vi "SetupDialog.vi"(8 "error in (no error)":errorcluster, 11 "Cluster in":T1 {"frequency" format="%0.2p"; "amplitude" format="%0.2p"; "phase" format="%.2p"; "sampling info"."Fs" format="%.2p"; "square wave duty cycle (%)" format="%0.2f"; "offset" format="%0.2p"}) -> (0 "error out":errorcluster, 3 "Cluster out":T1 {"frequency" format="%0.2p"; "amplitude" format="%0.2p"; "phase" format="%.2p"; "sampling info"."Fs" format="%.2p"; "square wave duty cycle (%)" format="%0.2f"; "offset" format="%0.2p"})   [LabVIEW 2022 SP3]
uses:
  MainBuf.ctl
panel:
  in  "frequency":dbl=10.0 format="%0.2p"
  in  "amplitude":dbl=1.0 format="%0.2p"
  in  "phase":dbl format="%.2p"
  in  "signal type":T2(ring)
  in  "sampling info":cluster{"Fs":dbl, "#s":dbl}={"Fs"=1024.0, "#s"=1024.0} {"Fs" format="%.2f"}
  in  "square wave duty cycle (%)":dbl=50.0 format="%0.2f"
  in  "offset":dbl format="%0.2p"
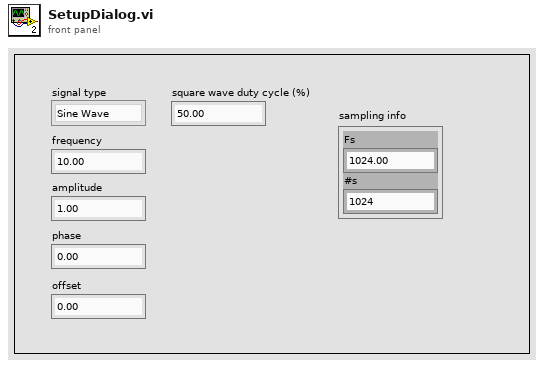
[diagram p1: front panel]
types:
  T1 = typedef "MainBuf.ctl" = cluster{"signal type":enum16{"Sine Wave", "Triangle Wave", "Square Wave", "Sawtooth Wave"}, "frequency":dbl, "amplitude":dbl, "phase":dbl, "offset":dbl, "square wave duty cycle (%)":dbl, "sampling info":cluster{"Fs":dbl, "#s":dbl}, "Reset":bool}
  T2 = enum16{"Sine Wave", "Triangle Wave", "Square Wave", "Sawtooth Wave"}
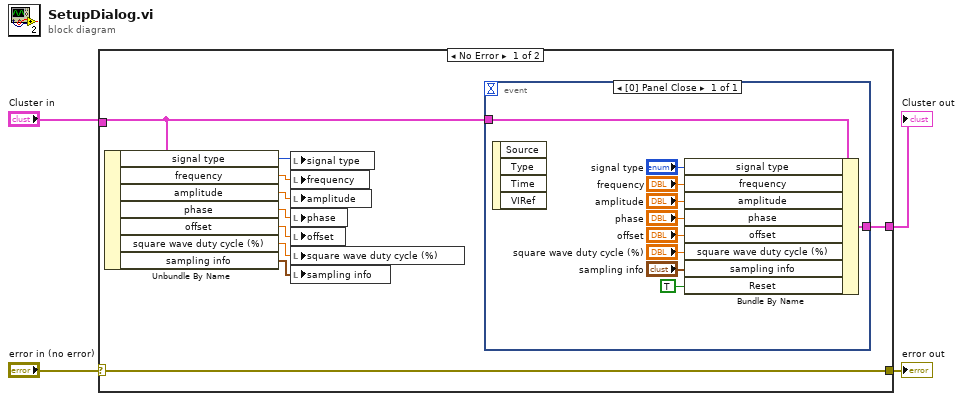
[diagram p0: block diagram]
diagram:
  n1 = case shown="No Error" "error in (no error)" {
    selector: "error in (no error)" -> [w13 w25]
    tunnel: "Cluster in" -> [w12 w26]
    tunnel: [w14 w26] -> w2
    tunnel: [w13 w25] -> w4
    frame No Error {
      n2 = Unbundle By Name(w12) -> ("signal type"=w11:T2, "frequency"=w10:dbl, "amplitude"=w9:dbl, "phase"=w8:dbl, "offset"=w7:dbl, "square wave duty cycle (%)"=w6:dbl, "sampling info"=w5:cluster{"Fs":dbl, "#s":dbl})
      n3 = local write "signal type"(w11) -> ()
      n4 = local write "frequency"(w10) -> ()
      n5 = local write "amplitude"(w9) -> ()
      n6 = local write "phase"(w8) -> ()
      n7 = local write "offset"(w7) -> ()
      n8 = local write "square wave duty cycle (%)"(w6) -> ()
      n9 = local write "sampling info"(w5) -> ()
      n10 = event shown="[0] Panel Close" {
        selector: _ -> [_]
        dyn-events: _ -> [_]
        timeout: _ -> [_]
        tunnel: [w24] -> w14
        tunnel: w12 -> [w15]
        event Panel Close {
          n11 = event-data() -> ()  [unwired: 1 in, 4 out]
          n12 = Bundle By Name(cluster=w15, "signal type"="signal type", "frequency"="frequency", "amplitude"="amplitude", "phase"="phase", "offset"="offset", "square wave duty cycle (%)"="square wave duty cycle (%)", "sampling info"="sampling info", "Reset"=TRUE) -> (w24:T1)
        }
      }
    }
    frame Error {
    }
  }
  "error out" <- w4
  "Cluster out" <- w2
